vi "SavedSettingsOpenAllVIs.vi"(6 "Tag":string, 8 "error in (no error)":errorcluster, 9 "Dummy prefix":string="???? ", 10 "Saved Settings":refnum<vi>, 11 "Control Tree in":refnum<vi>) -> (0 "error out":errorcluster, 3 "Control Tree out":refnum<vi>)   [LabVIEW 2020]
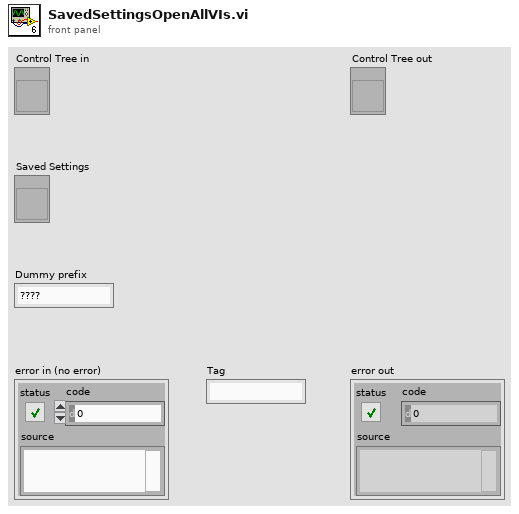
[diagram p1: front panel]
types:
  T1 = enum32{"Invalid", "Standard", "Closed", "Hidden", "Minimized", "Maximized"}
  T2 = cluster{"Closed Nodes":string[], "Selection":string[], "Defer Panel Update":bool}
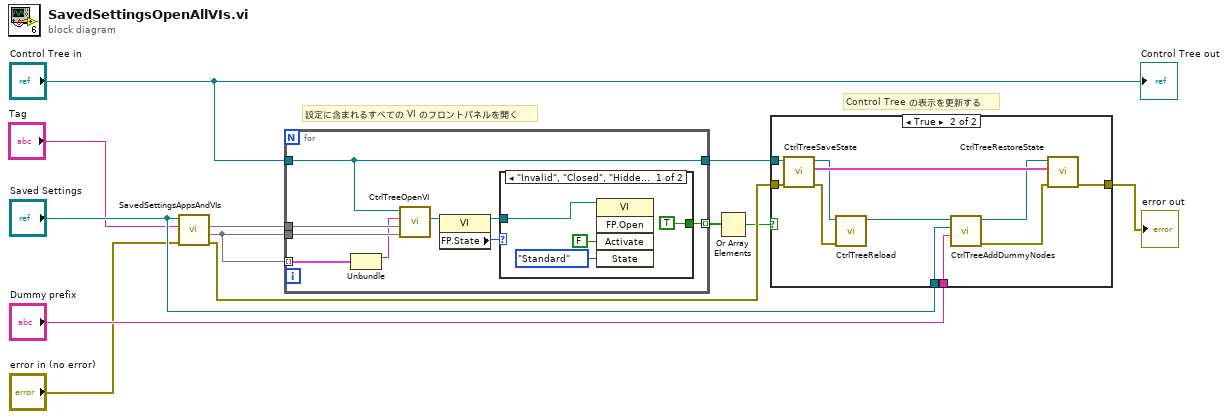
[diagram p0: block diagram]
diagram:
  # "Control Tree の表示を更新する"
  # "設定に含まれるすべての VI のフロントパネルを開く"
  n1 = call "SavedSettingsAppsAndVIs.vi"("error in (no error)"="error in (no error)", "Tag"="Tag", "SavedSettings in"="Saved Settings") -> ("error out"=w5:errorcluster, "VIs"=w10:map{string, string}, "Apps"=w11:map{string, string})  [unwired: 5 in, 1 out]
  n2 = for {
    tunnel: "Control Tree in" -> [w17]
    tunnel: w10 -> [w21]
    tunnel: w11 -> [w20]
    tunnel: w10 -> [w19] mode=indexing
    tunnel: [w17] -> w9
    tunnel: [w13] -> w2 mode=indexing
    n3 = Unbundle(w19) -> (w18:string)  [unwired: 1 out]
    n4 = call "CtrlTreeOpenVI.vi"("VIs"=w21, "Apps"=w20, "Tag"=w18, "ControlTree in"=w17) -> ("VI ref"=w16:refnum<vi>)  [unwired: 5 in, 2 out]
    n5 = property class="VI"(reference=w16) -> (reference out=w15:refnum<vi>, "FP.State"=w14:T1)  [unwired: 1 in, 1 out]
    n6 = case shown="\"Invalid\", \"Closed\", \"Hidden\"" w14 {
      tunnel: w15 -> [w23 _]
      tunnel: [TRUE _] -> w13
      frame "Invalid", "Closed", "Hidden" {
        n7 = invoke class="VI" method="FP.Open"(reference=w23, "Activate"=FALSE ("Activate?"), "State"=T1."Standard") -> ()  [unwired: 2 in, 5 out]
      }
      frame Default {
      }
    }
  }
  n8 = Or Array Elements(Boolean array=w2) -> (logical OR=w1:bool)
  n9 = case shown="True" w1 {
    tunnel: w9 -> [_ w37]
    tunnel: "Saved Settings" -> [_ w35]
    tunnel: "Dummy prefix" -> [_ w34]
    tunnel: w5 -> [w26 w28]
    tunnel: [w26 w27] -> w4
    frame False {
    }
    frame True {
      n10 = call "CtrlTreeSaveState.vi"("error in (no error)"=w28, "TreeControl in"=w37) -> ("error out"=w32:errorcluster, "State"=w36:T2, "TreeControl out"=w33:refnum<vi>)  [unwired: 7 in]
      n11 = call "CtrlTreeReload.vi"("error in (no error)"=w32, "TreeControl in"=w33) -> ("TreeControl out"=w31:refnum<vi>)  [unwired: 9 in]
      n12 = call "CtrlTreeAddDummyNodes.vi"("Dummy prefix"=w34, "SavedSettings in"=w35, "TreeControl in"=w31) -> ("error out"=w29:errorcluster, "TreeControl out"=w30:refnum<vi>)  [unwired: 7 in]
      n13 = call "CtrlTreeRestoreState.vi"("error in (no error)"=w29, "State"=w36, "TreeControl in"=w30) -> ("error out"=w27:errorcluster)  [unwired: 7 in, 1 out]
    }
  }
  "error out" <- w4
  "Control Tree out" <- "Control Tree in"
